vi "create_corewebview2.vi"(8 "error in":errorcluster, 11 "WebView2":refnum<k24>) -> (0 "error out":errorcluster, 3 "CoreWebView2":refnum<k24>)   [LabVIEW 2020, in "simple_html_chat_ui.lvclass"]
uses:
  simple_html_chat_ui.lvclass
  D:/petwork/labview-llm-libraries/src/user_interfaces/simple_html_chat_ui/assembly_support/Microsoft.Web.WebView2.WinForms.dll
  assembly_support/Microsoft.Web.WebView2.WinForms.dll
  D:/petwork/labview-llm-libraries/src/user_interfaces/simple_html_chat_ui/assembly_support/Microsoft.Web.WebView2.Core.dll
  assembly_support/Microsoft.Web.WebView2.Core.dll
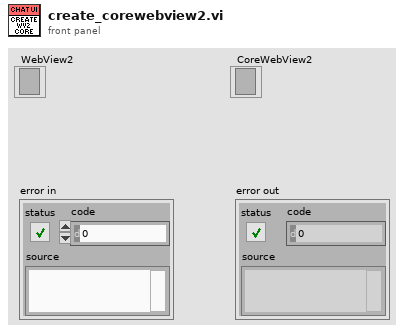
[diagram p1: front panel]
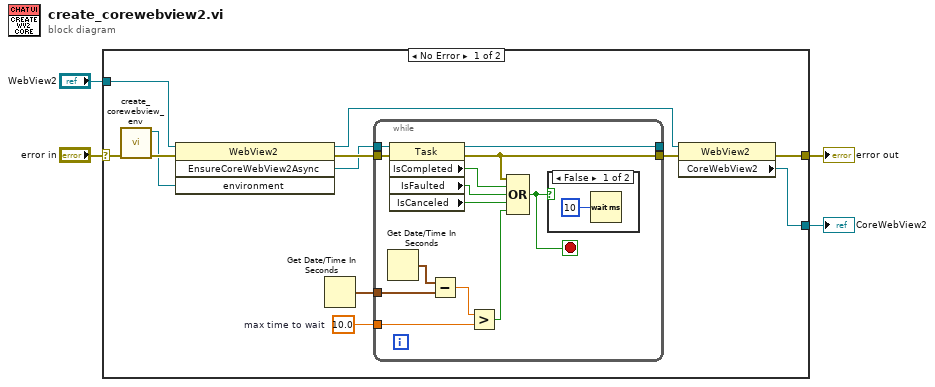
[diagram p0: block diagram]
diagram:
  n1 = case shown="No Error" "error in" {
    selector: "error in" -> [w9 w31]
    tunnel: "WebView2" -> [w10 _]
    tunnel: [w6 w31] -> w2
    tunnel: [w5 _] -> w1
    frame No Error {
      w7 = 10.0  # max time to wait
      n2 = call "create_corewebview_env.vi"("error in"=w9) -> ("error out"=w16:errorcluster, "Environment"=w15:refnum<k24>)  [unwired: 9 in]
      n3 = invoke class="WebView2" method="EnsureCoreWebView2Async"(reference=w10, error in=w16, "environment"=w15) -> (reference out=w11:refnum<k24>, error out=w14:errorcluster, "EnsureCoreWebView2Async"=w13:refnum<k24>)  [unwired: 1 in, 1 out]
      n4 = Get Date/Time In Seconds() -> (seconds since 1Jan1904=w8:timestamp)
      n5 = while {
        tunnel: w13 -> [w29]
        tunnel: w14 -> [w28]
        tunnel: [w27] -> _
        tunnel: [w26] -> w12
        tunnel: w8 -> [w20]
        tunnel: w7 -> [w18]
        stop <- w23 stop-if-true
        n6 = Get Date/Time In Seconds() -> (seconds since 1Jan1904=w21:timestamp)
        n7 = property class="Task"(reference=w29, error in=w28) -> (reference out=w27:refnum<k24>, error out=w26:errorcluster, "IsCompleted"=w22:bool, "IsFaulted"=w25:bool, "IsCanceled"=w24:bool)
        n8 = Subtract(x=w21, y=w20) -> (x-y=w19:dbl)
        n9 = Greater?(x=w19, y=w18) -> (0:w17:bool)
        n10 = Compound Arithmetic op=OR(w26, w22, w25, w24, w17) -> (w23:bool)
        n11 = case shown="False" w23 {
          frame False {
            n12 = Wait (ms)(milliseconds to wait=u32 10) -> ()  [unwired: 1 out]
          }
          frame True {
          }
        }
      }
      n13 = property class="WebView2"(reference=w11, error in=w12) -> (error out=w6:errorcluster, "CoreWebView2"=w5:refnum<k24>)  [unwired: 1 out]
    }
    frame Error {
    }
  }
  "error out" <- w2
  "CoreWebView2" <- w1
